vi "bundle-unbundle-names.vi"() -> ()   [LabVIEW 2025]
panel:
  out "Name":string
  out "size":u32
  out "Elements in array":u32
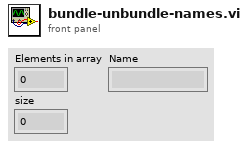
[diagram p1: front panel]
types:
  T1 = cluster{"Name":string, "Elements in array":u32, "size":u32}
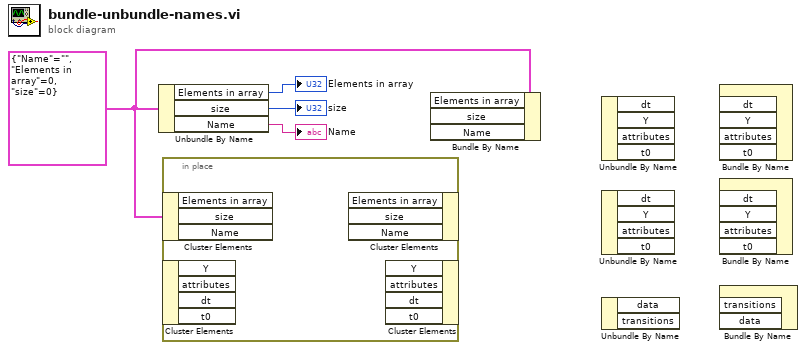
[diagram p0: block diagram]
diagram:
  w1 = T1 {"Name"="", "Elements in array"=0, "size"=0} ("input cluster")
  n1 = Unbundle By Name(w1) -> ("Elements in array"=→"Elements in array":u32, "size"=→"size":u32, "Name"=→"Name":string)
  n2 = in-place {
    n3 = in-place-cluster #1 ("Unbundle / Bundle Elements")(w1) -> ()  [unwired: 3 out]
    n4 = in-place-cluster #2 ("Waveform Unbundle / Bundle Elements")() -> ()  [unwired: 1 in, 4 out]
    n5 = in-place-cluster #1() -> ()  [unwired: 3 in, 1 out]
    n6 = in-place-cluster #2() -> ()  [unwired: 4 in, 1 out]
  }
  n7 = Bundle By Name(cluster=w1) -> ()  [unwired: 3 in, 1 out]
  n8 = Unbundle By Name() -> ()  [unwired: 1 in, 4 out]
  n9 = Unbundle By Name ("Get Waveform Components")() -> ()  [unwired: 1 in, 4 out]
  n10 = Unbundle By Name ("Get Digital Data Components")() -> ()  [unwired: 1 in, 2 out]
  n11 = Bundle By Name() -> ()  [unwired: 5 in, 1 out]
  n12 = Bundle By Name() -> ()  [unwired: 5 in, 1 out]
  n13 = Bundle By Name() -> ()  [unwired: 3 in, 1 out]
